vi "Close Connection.vi"(8 "error in (no error)":errorcluster, 11 "Network Stream in":refnum<class "Network Stream.lvclass">) -> (0 "error out":errorcluster, 3 "Network Stream out":refnum<class "Network Stream.lvclass">)   [LabVIEW 2019, in "Network Stream.lvlib" / "Network Stream.lvclass"]
uses:
  Network Stream.lvclass
  Network Stream.lvclass/Network Stream.ctl
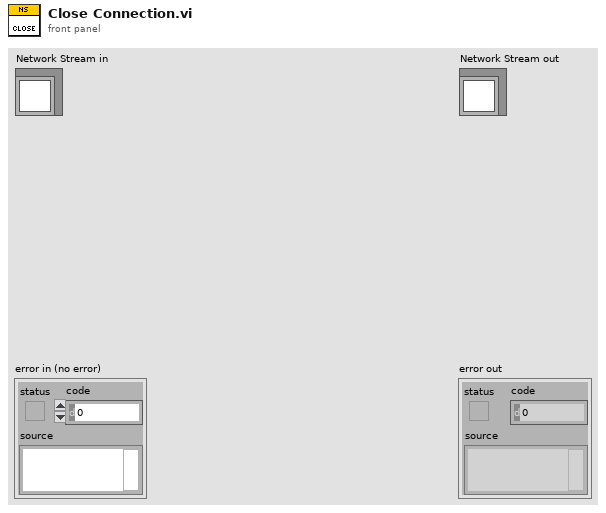
[diagram p1: front panel]
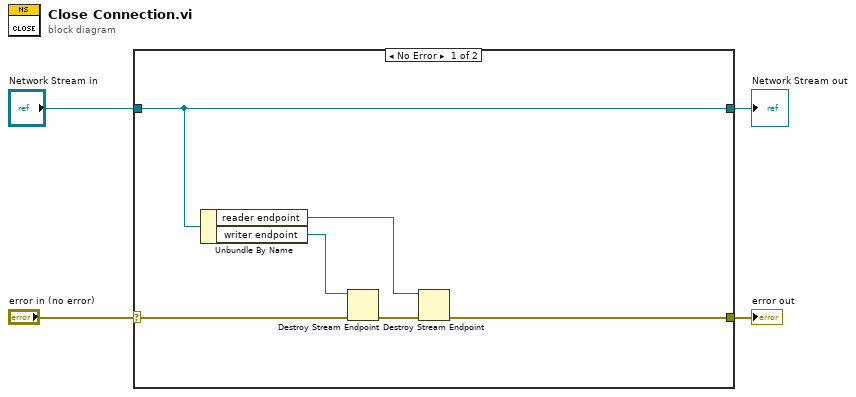
[diagram p0: block diagram]
diagram:
  n1 = case shown="No Error" "error in (no error)" {
    selector: "error in (no error)" -> [w8 w12]
    tunnel: [w7 w12] -> w3
    tunnel: [w5 w11] -> w1
    tunnel: "Network Stream in" -> [w5 w11]
    frame No Error {
      n2 = Unbundle By Name(w5) -> ("reader endpoint"=w9:refnum<k21>, "writer endpoint"=w10:refnum<k21>)
      n3 = Destroy Stream Endpoint(8:w8, 11:w10) -> (0:w6:errorcluster)
      n4 = Destroy Stream Endpoint(8:w6, 11:w9) -> (0:w7:errorcluster)
    }
    frame Error {
    }
  }
  "error out" <- w3
  "Network Stream out" <- w1
